vi "Get All Delays.vi"(0 "VISA Ref":refnum<visa-resource-name>) -> (4 "VISA Ref Dup":refnum<visa-resource-name>, 15 "Delays (steps)":dbl[](array[numeric]))   [LabVIEW 2016]
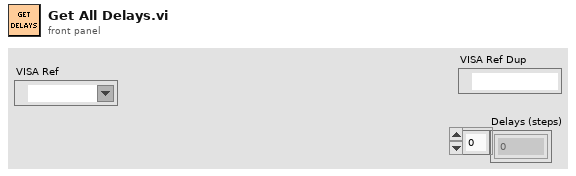
[diagram p1: front panel]
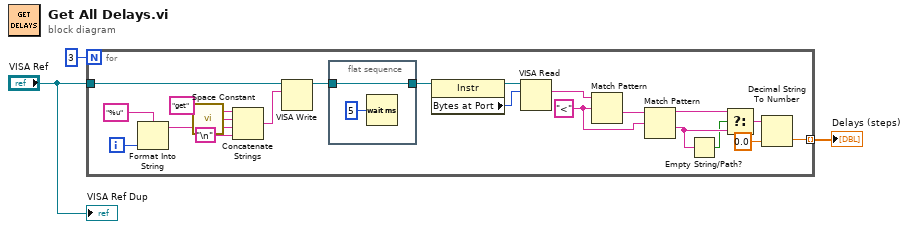
[diagram p0: block diagram]
diagram:
  n1 = for {
    N: 3 -> [_]
    tunnel: [w6] -> w1 mode=indexing
    tunnel: "VISA Ref" -> [w5]
    i -> [w24]
    w10 = "<" ("regular expression")
    n2 = Format Into String(format string="%u", w24) -> (resulting string=w21:string)  [unwired: 2 in, 1 out]
    n3 = call <vilib>:"Space Constant.vi"() -> ("String"=w19:string)
    n4 = Concatenate Strings("get", w19, w21, "\n") -> (w18:string)
    n5 = VISA Write(VISA resource name=w5, write buffer=w18) -> (VISA resource name out=w17:refnum<visa-resource-name>)  [unwired: 1 in, 2 out]
    n6 = flat-sequence {
      tunnel: w17 -> [w25]
      tunnel: [w25] -> w16
      frame #0 {
        n7 = Wait (ms)(milliseconds to wait=u32 5) -> ()  [unwired: 1 out]
      }
    }
    n8 = property class="Instr"(reference=w16) -> (reference out=w15:refnum<visa-resource-name>, "Bytes at Port"=w14:u32)  [unwired: 1 in, 1 out]
    n9 = VISA Read(VISA resource name=w15, byte count=w14) -> (read buffer=w8:string)  [unwired: 1 in, 3 out]
    n10 = Match Pattern(string=w8, regular expression=w10) -> (after substring=w9:string)  [unwired: 1 in, 3 out]
    n11 = Match Pattern(string=w9, regular expression=w10) -> (before substring=w13:string, after substring=w12:string)  [unwired: 1 in, 2 out]
    n12 = Empty String/Path?(string/path=w12) -> (empty?=w11:bool)
    n13 = Select(t=w13, s=w11, f=w12) -> (s? t:f=w7:string)
    n14 = Decimal String To Number(string=w7, default (0L)=0.0) -> (number=w6:dbl)  [unwired: 1 in, 1 out]
  }
  "Delays (steps)" <- w1
  "VISA Ref Dup" <- "VISA Ref"
